vi "M00 TV.vi"(11 "NXT/EV3":T1) -> (3 "EV3 out":T1)   [LabVIEW 2016]
uses:
  <vilib>/NXT/Subs/LVHSConnector.ctl
  <vilib>/NXT/LegoClasses/BrickReference/BrickReference.lvclass
  <vilib>/NXT/Dual Mode Library/Waits/Wait_Num.vi
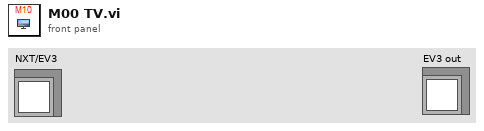
[diagram p1: front panel]
types:
  T1 = typedef "LVHSConnector.ctl" = refnum<class "BrickReference.lvclass">
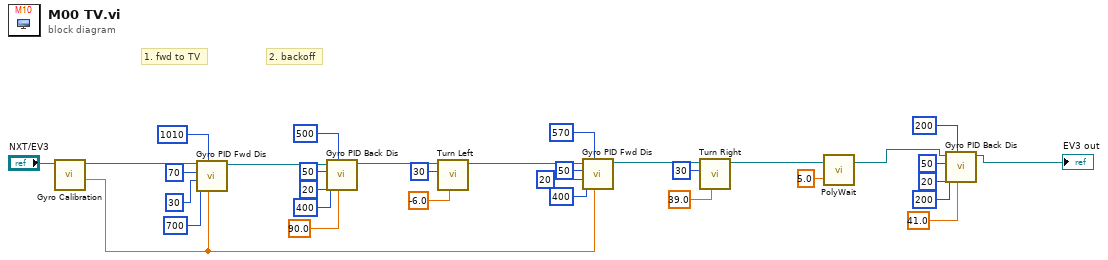
[diagram p0: block diagram]
diagram:
  # "2. backoff"
  # "1. fwd to TV"
  n1 = call "Gyro Calibration.vi"("NXT/EV3"="NXT/EV3") -> ("Degrees"=w17:sgl, "NXT/EV3"=w23:T1)  [unwired: 6 in, 1 out]
  n2 = call "Gyro PID Fwd Dis.vi"("Target angle"=w17, "Threshold to stop"=1010, "Threshold to slow"=700, "Min. speed"=30, "Max. speed"=70, "EV3 in"=w23) -> ("EV3 out"=w28:T1)  [unwired: 5 in]
  n3 = call "Gyro PID Back Dis.vi"("Target angle"=sgl 90.0, "Threshold to stop"=500, "Threshold to slow"=400, "Min. speed"=20, "Max. speed"=50, "EV3 in"=w28) -> ("EV3 out"=w15:T1)  [unwired: 5 in]
  n4 = call "Turn Left.vi"("Turning angle"=sgl -6.0, "Motor B (right)"=i8 30, "EV3 in"=w15) -> ("EV3 out"=w12:T1)  [unwired: 8 in]
  n5 = call "Gyro PID Fwd Dis.vi"("Target angle"=w17, "Threshold to stop"=570, "Threshold to slow"=400, "Min. speed"=20, "Max. speed"=50, "EV3 in"=w12) -> ("EV3 out"=w16:T1)  [unwired: 5 in]
  n6 = call "Turn Right.vi"("Turning angle"=sgl 39.0, "Motor B (right)"=i8 30, "EV3 in"=w16) -> ("EV3 out"=w8:T1)  [unwired: 8 in]
  n7 = call-poly <vilib>:"PolyWait.vi"("Time (1 sec)"=sgl 5.0, "NXT/EV3"=w8) -> ("NXT/EV3"=w2:T1)  [unwired: 2 in]
  n8 = call "Gyro PID Back Dis.vi"("Target angle"=sgl 41.0, "Threshold to stop"=200, "Threshold to slow"=200, "Min. speed"=20, "Max. speed"=50, "EV3 in"=w2) -> ("EV3 out"=→"EV3 out":T1)  [unwired: 5 in]
